vi "Updater Convert TDMS Test Runs 4.3 to 5.0.vi"(6 "New TDMS File In":refnum<k34>, 7 "Map IndexName to FieldId":T1(array[cluster]), 8 "error in (no error)":errorcluster, 9 "Test Type":string, 10 "Group Name In":string, 11 "Source TDMS File In":refnum<k34>) -> (0 "error out":errorcluster, 2 "Group Name Out":string, 3 "Source TDMS File Out":refnum<k34>, 4 "New TDMS File Out":refnum<k34>)   [LabVIEW 2011]
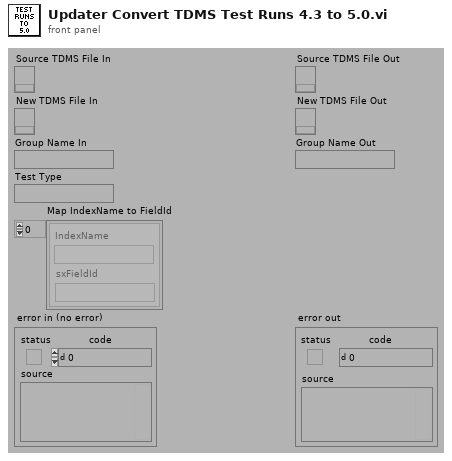
[diagram p1: front panel]
types:
  T1 = cluster{"IndexName":string, "sxFieldId":string}[]
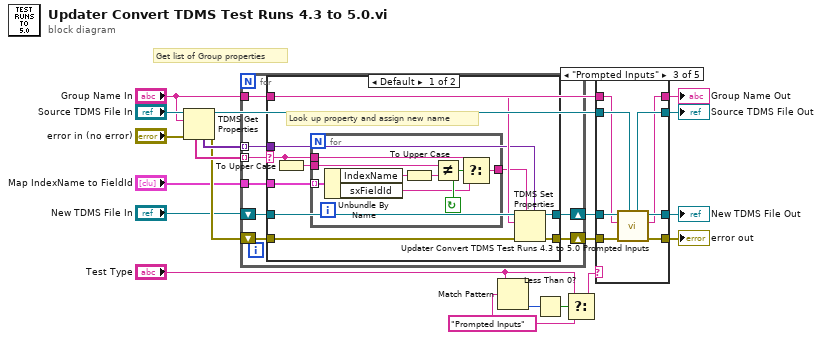
[diagram p0: block diagram]
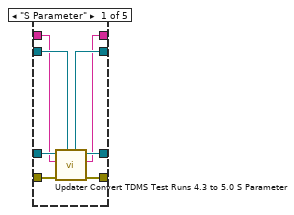
[diagram p3: hidden frame]
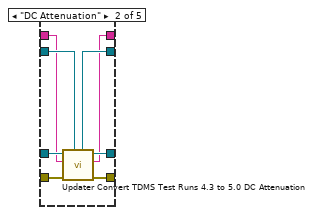
[diagram p4: hidden frame]
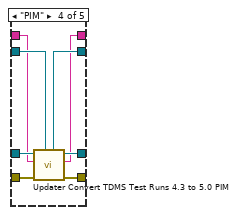
[diagram p5: hidden frame]
diagram:
  w3 = "Prompted Inputs" ("element")
  # "Get list of Group properties"
  n1 = TDMS Get Properties(8:"error in (no error)", 10:"Group Name In", 11:"Source TDMS File In") -> (0:w14:errorcluster, 3:w7:refnum<k34>, 4:w16:variant[], 6:w15:string[])  [unwired: 5 out]
  n2 = for {
    shift-right: [w27] -> w12
    shift-left: w14 -> [w28]
    tunnel: "Group Name In" -> [w25]
    tunnel: w15 -> [w24] mode=indexing
    tunnel: w16 -> [w23] mode=indexing
    tunnel: "Map IndexName to FieldId" -> [w22]
    shift-right: [w21] -> w8
    shift-left: "New TDMS File In" -> [w26]
    n3 = case shown="Default" w24 {
      selector: w24 -> [w32 _]
      tunnel: w28 -> [w35 w48]
      tunnel: [w38 w48] -> w27
      tunnel: w26 -> [w37 w47]
      tunnel: w25 -> [w36 _]
      tunnel: w23 -> [w34 _]
      tunnel: w22 -> [w33 _]
      tunnel: [w30 w47] -> w21
      frame Default {
        # "Look up property and assign new name"
        n4 = To Upper Case(1:w32) -> (0:w29:string)
        n5 = for {
          tunnel: w33 -> [w46] mode=indexing
          tunnel: w32 -> [w44]
          tunnel: [w41] -> w31
          tunnel: w29 -> [w45]
          stop <- w43 continue-if-true
          n6 = Unbundle By Name(w46) -> ("IndexName"=w40:string, "sxFieldId"=w42:string)
          n7 = To Upper Case(1:w40) -> (0:w39:string)
          n8 = Not Equal?(x=w45, y=w39) -> (x != y?=w43:bool)
          n9 = Select(t=w44, s=w43, f=w42) -> (s? t:f=w41:string)
        }
        n10 = TDMS Set Properties(5:w34, 7:w31, 8:w35, 10:w36, 11:w37) -> (0:w38:errorcluster, 3:w30:refnum<k34>)  [unwired: 3 out]
      }
      frame "Company", "Data_File", "datatype", "Description", "End_Timestamp", "index", "maximum", "minimum", "Model_Number", "Name", "NI_channellength", "NI_DataType", "Operator", "registertxt1", "Serial_Number", "Start_Timestamp", "Step_Number", "Step_Tag", "Test_Run", "Test_Sequence", "Test_Station", "Test_Station_Name", "Test_Status", "Test_Type", "Test_Version", "wf_increment", "wf_samples", "wf_start_offset", "wf_start_time" {
        # "Process only Custom Fields as the NI specific properties,\ncommon properties, and test specific properties are not\nprocessed here."
      }
    }
  }
  n11 = Match Pattern(string="Test Type", regular expression=w3) -> (offset past match=w5:i32)  [unwired: 4 out]
  n12 = Less Than 0?(x=w5) -> (x < 0?=w4:bool)
  n13 = Select(t="Test Type", s=w4, f=w3) -> (s? t:f=w1:string)
  n14 = case shown="\"Prompted Inputs\"" w1 {
    tunnel: w7 -> [w54 w62 w70 w78 w84]
    tunnel: [w53 w61 w69 w77 w84] -> w20
    tunnel: "Group Name In" -> [w50 w58 w66 w74 w83]
    tunnel: [w49 w57 w65 w73 w83] -> w19
    tunnel: w8 -> [w55 w63 w71 w79 w82]
    tunnel: [w52 w60 w68 w76 w82] -> w18
    tunnel: [w51 w59 w67 w75 w81] -> w17
    tunnel: w12 -> [w56 w64 w72 w80 w81]
    frame "S Parameter" {
      n15 = call "Updater Convert TDMS Test Runs 4.3 to 5.0 S Parameter.vi"("Source TDMS File In"=w54, "error in (no error)"=w56, "Group Name In"=w50, "New TDMS File In"=w55) -> ("error out"=w51:errorcluster, "Group Name Out"=w49:string, "New TDMS File Out"=w52:refnum<k34>, "Source TDMS File Out"=w53:refnum<k34>)  [unwired: 2 in, 2 out]
    }
    frame "DC Attenuation" {
      n16 = call "Updater Convert TDMS Test Runs 4.3 to 5.0 DC Attenuation.vi"("Source TDMS File In"=w62, "error in (no error)"=w64, "Group Name In"=w58, "New TDMS File In"=w63) -> ("error out"=w59:errorcluster, "Group Name Out"=w57:string, "New TDMS File Out"=w60:refnum<k34>, "Source TDMS File Out"=w61:refnum<k34>)  [unwired: 4 out]
    }
    frame "Prompted Inputs" {
      n17 = call "Updater Convert TDMS Test Runs 4.3 to 5.0 Prompted Inputs.vi"("Source TDMS File In"=w70, "error in (no error)"=w72, "Group Name In"=w66, "New TDMS File In"=w71) -> ("error out"=w67:errorcluster, "Group Name Out"=w65:string, "New TDMS File Out"=w68:refnum<k34>, "Source TDMS File Out"=w69:refnum<k34>)  [unwired: 4 out]
    }
    frame "PIM" {
      n18 = call "Updater Convert TDMS Test Runs 4.3 to 5.0 PIM.vi"("Source TDMS File In"=w78, "error in (no error)"=w80, "Group Name In"=w74, "New TDMS File In"=w79) -> ("error out"=w75:errorcluster, "Group Name Out"=w73:string, "New TDMS File Out"=w76:refnum<k34>, "Source TDMS File Out"=w77:refnum<k34>)  [unwired: 4 out]
    }
    frame Default {
    }
  }
  "error out" <- w17
  "Group Name Out" <- w19
  "Source TDMS File Out" <- w20
  "New TDMS File Out" <- w18
